vi "CLC_GEN4_L2_InPhaseCal.vi"() -> ()   [LabVIEW 2023, in "Clover_Cell.lvlib"]
uses:
  Clover_Cell.lvlib
  lib/Anritsu Signal Analyzer Series/Anritsu Signal Analyzer Series.lvlib
  lib/ELTA/ELTA.lvlib
  <vilib>/Utility/file.llb/Write Delimited Spreadsheet (DBL).vi
panel:
  out "Check Ref. Ch.":i32[][](array[numeric])
  in  "Dual_Ch.???":bool=TRUE
  in  "Single_Channel_Phase_Sweep":bool
  in  "Polarity":u16(ring) items=["V", "H"]
  in  "AvgTimes":i32=3
  in  "TRXmode":u16(ring)=1 items=["Rx"=2, "Tx"=1]
  in  "CenterFreq(GHz)":dbl=27.0
  in  "VISA resource name":refnum<visa-resource-name>="TCPIP0::192.168.100.230::inst0::INSTR"
  out "Channel":i32=63
  out "Operating \nChannel(s)":bool[][](array[boolean])
  out "FileNAME_Dual":string
  out "FileNAME_Single":string
  out "PhaseStep":i32=63
  out "OK?":bool
  out "output cluster":T1={"address"="192.168.100.111", "remote port or service name"=5025, "timeout ms (60000)"=10000}
  out "SA1":dbl[](graph)
  out "trmode":u16=1
  out "TotalTime":dbl format="%.2f"
  out "StopTime":timestamp=timestamp(3663835912.033212 s since 1904-01-01)
  out "Data":dbl[][](array[numeric])
  out "StartTime":timestamp=timestamp(3663835741.875155 s since 1904-01-01)
  out "error out":errorcluster
  out "CurrentData":dbl[](array[numeric])
  out "Duration":dbl
  # "Setting"
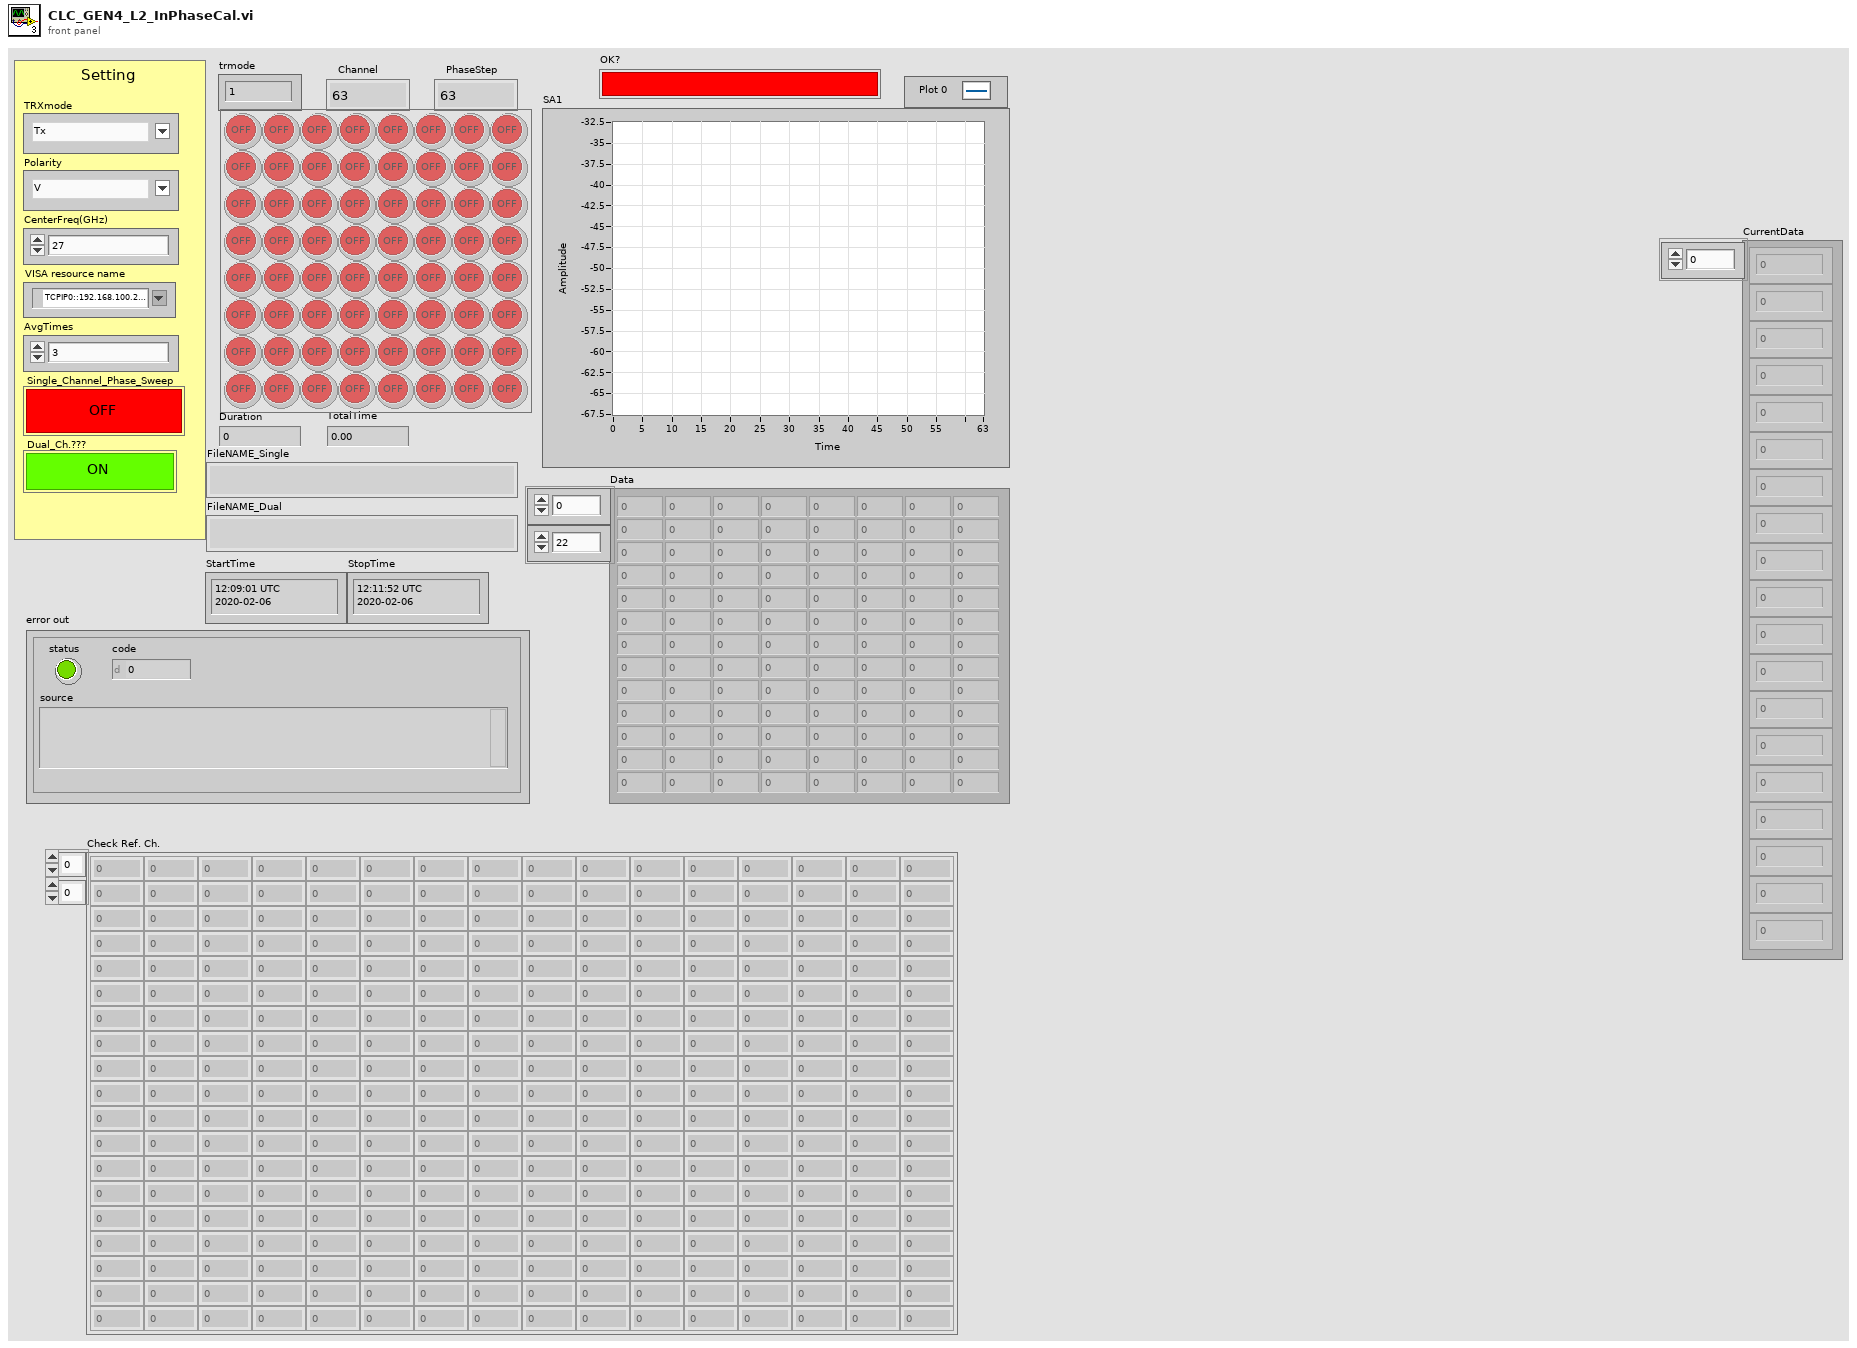
[diagram p1: front panel]
types:
  T1 = cluster{"address":string, "remote port or service name":u16, "timeout ms (60000)":i32}
  T2 = cluster{"Mode":u16, "Polarity":u16, "CH_ON/OFF":u16, "Channel":i32, "Gain":i32, "Phase":i32}
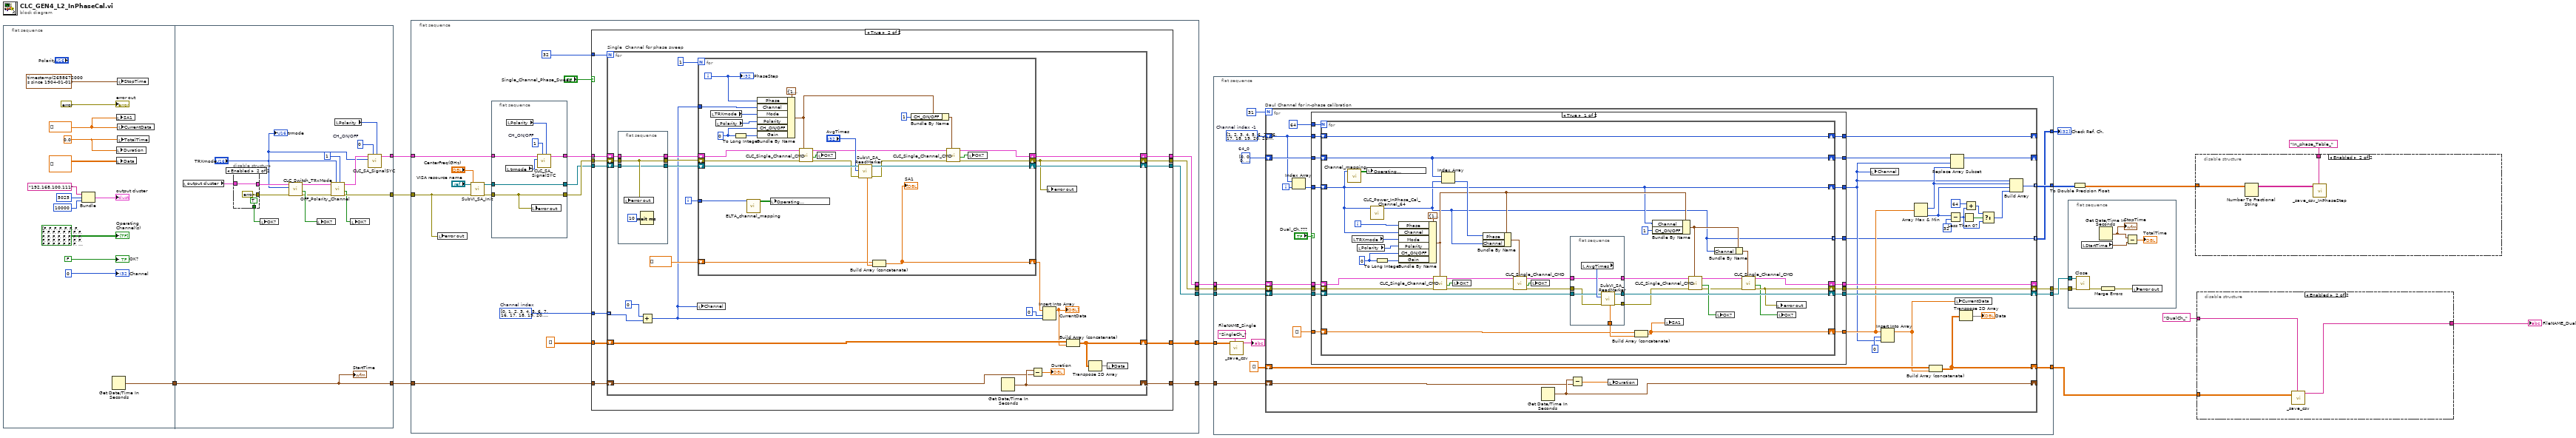
[diagram p0: block diagram]
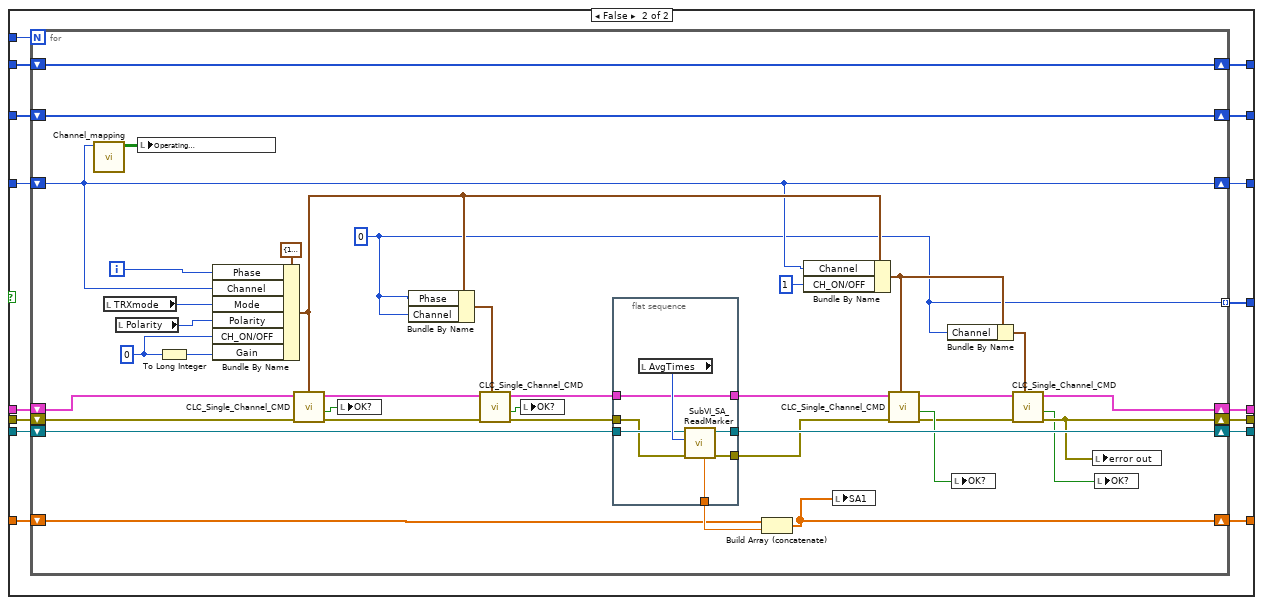
[diagram p2: hidden frame]
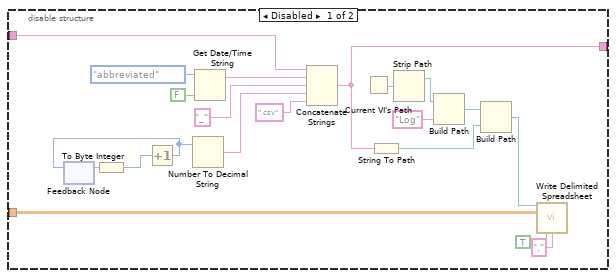
[diagram p4: hidden frame]
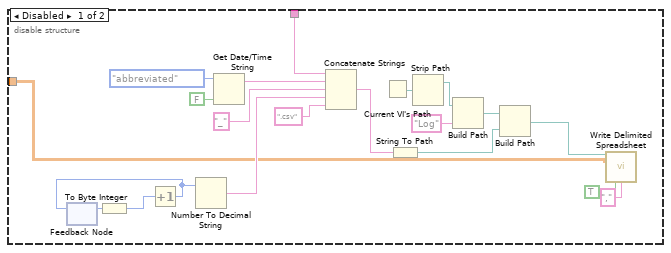
[diagram p5: hidden frame]
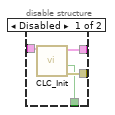
[diagram p6: hidden frame]
diagram:
  n1 = flat-sequence {
    tunnel: [w19] -> w4
    tunnel: w4 -> [w35]
    tunnel: [w38] -> w5
    tunnel: [w42] -> w8
    tunnel: [w35] -> w18
    frame #0 {
      w23 = dbl[] []
      w26 = 0.0 ("TotalTime")
      n2 = Bundle("address"="192.168.100.111", "remote port or service name"=u16 5025, "timeout ms (60000)"=10000) -> (→"output cluster":T1)  [unwired: 1 in]
      n3 = Get Date/Time In Seconds() -> (seconds since 1Jan1904=w19:timestamp)
      n4 = local write "SA1"(w23) -> ()
      n5 = local write "Duration"(w26) -> ()
      n6 = local write "Data"(dbl[][] []) -> ()
      n7 = local write "StopTime"(timestamp(2658672000.001 s since 1904-01-01) ("StopTime")) -> ()
      n8 = local write "CurrentData"(w23) -> ()
      n9 = local write "TotalTime"(w26) -> ()
      "error out" <- errorcluster {"status"=FALSE, "code"=0, "source"=""} ("error out")
      "Operating \nChannel(s)" <- bool[][] [[FALSE, FALSE, FALSE, FALSE, FALSE, FALSE, FALSE, FALSE], [FALSE, FALSE, FALSE, FALSE, FALSE, FALSE, FALSE, FALSE], [FALSE, FALSE, FALSE, FALSE, FALSE, FALSE, FALSE, FALSE], [FALSE, FALSE, FALSE, FALSE, FALSE, FALSE, FALSE, FALSE], [FALSE, FALSE, FALSE, FALSE, FALSE, FALSE, FALSE, FALSE], [FALSE, FALSE, FALSE, FALSE, FALSE, FALSE, FALSE, FALSE], [FALSE, FALSE, FALSE, FALSE, FALSE, FALSE, FALSE, FALSE], [FALSE, FALSE, FALSE, FALSE, FALSE, FALSE, FALSE, FALSE]] ("Operating \nChannel(s)")
      "Channel" <- 0 ("Channel")
      "OK?" <- FALSE ("OK?")
    }
    frame #1 {
      w37 = u16 0  # CH_ON/OFF
      n10 = local read "output cluster"() -> (w47:T1)
      n11 = disable-structure shown="Enabled" {
        disable-tunnel: w47 -> [w51 w54]
        disable-tunnel: [w50 w54] -> w46
        disable-tunnel: [w49 errorcluster {"status"=FALSE, "code"=0, "source"=""} ("error in (no error)")] -> w44
        disable-tunnel: [w48 TRUE ("OK?")] -> w36
        frame Disabled {
          n12 = call "CLC_Init.vi"("TCPIPin"=w51) -> ("error out"=w49:errorcluster, "Status"=w48:bool, "TCPIPin 2"=w50:T1)  [unwired: 8 in]
        }
        frame Enabled {
        }
      }
      n13 = local write "OK?"(w36) -> ()
      n14 = call "CLC_Switch_TRxMode.vi"("error in (no error)"=w44, "Text Ring"="TRXmode", "TCPIPin"=w46) -> ("error out"=w43:errorcluster, "OK?"=w45:bool, "TCPIPin 2"=w41:T1)  [unwired: 6 in]
      n15 = local write "OK?"(w45) -> ()
      n16 = call "OFF_Polarity_Channel.vi"("CH_ON:0/OFF:1"=u16 1, "Mode"="TRXmode", "error in"=w43, "TCPIPin"=w41) -> ("error out"=w42:errorcluster, "OK?"=w40:bool, "TCPIPout"=w39:T1)  [unwired: 5 in]
      n17 = local read "Polarity"() -> (w33:u16)
      n18 = local write "OK?"(w40) -> ()
      n19 = call "CLC_SA_SignalSYC.vi"("Polarity"=w33, "CH_ON/OFF"=w37, "Mode"="TRXmode", "TCPIPin"=w39) -> ("TCPIPout"=w38:T1)  [unwired: 7 in]
      "StartTime" <- w35
      "trmode" <- "TRXmode"
    }
  }
  n20 = flat-sequence {
    tunnel: w18 -> [w71]
    tunnel: [w70] -> w17
    tunnel: [w69] -> w16
    tunnel: [w68] -> w15
    tunnel: [w67] -> w9
    tunnel: w8 -> [w65]
    tunnel: w5 -> [w60]
    tunnel: [w55] -> w3
    frame #0 {
      w62 = i32[] [0, 1, 2, 3, 4, 5, 6, 7, 16, 17, 18, 19, 20, 21, 22, 23, 32, 33, 34, 35, 36, 37, 38, 39, 48, 49, 50, 51, 52, 53, 54, 55]  # Channel index
      n21 = local write "error out"(w65) -> ()
      n22 = call "SubVI_SA_Init.vi"("error in (no error)"=w65, "CenterFreq(GHz) 2"="CenterFreq(GHz)", "VISA resource name"="VISA resource name") -> ("error out 2"=w66:errorcluster, "VISA resource name out"=w59:refnum<visa-resource-name>)  [unwired: 6 in, 1 out]
      n23 = flat-sequence {
        tunnel: w66 -> [w152]
        tunnel: [w152] -> w61
        tunnel: w60 -> [w150]
        tunnel: w59 -> [w151]
        tunnel: [w151] -> w58
        tunnel: [w149] -> w57
        frame #0 {
          w148 = u16 1  # CH_ON/OFF
          n24 = local read "trmode"() -> (w146:u16)
          n25 = local read "Polarity"() -> (w147:u16)
          n26 = local write "error out"(w152) -> ()
          n27 = call "CLC_SA_SignalSYC.vi"("Polarity"=w147, "CH_ON/OFF"=w148, "Mode"=w146, "TCPIPin"=w150) -> ("TCPIPout"=w149:T1)  [unwired: 7 in]
        }
      }
      n28 = case shown="True" "Single_Channel_Phase_Sweep" {
        tunnel: [w75 w90] -> w55
        tunnel: 32 -> [_ w89]
        tunnel: w71 -> [w74 w88]
        tunnel: [w76 w87] -> w70
        tunnel: [w77 w86] -> w69
        tunnel: [w78 w85] -> w68
        tunnel: [w74 w84] -> w67
        tunnel: dbl[][] [] -> [w75 w83]
        tunnel: w62 -> [_ w82]
        tunnel: w61 -> [w77 w81]
        tunnel: w58 -> [w76 w80]
        tunnel: w57 -> [w78 w79]
        frame False {
        }
        frame True {
          n29 = for "Single  Channel for phase sweep" {
            N: w89 -> [_]
            shift-right: [w114] -> w85
            shift-left: w79 -> [w98]
            shift-right: [w108] -> w86
            shift-left: w81 -> [w100]
            shift-right: [w112] -> w87
            shift-left: w80 -> [w97]
            shift-right: [w106] -> w90
            shift-left: w83 -> [w107]
            shift-right: [w110] -> w84
            shift-left: w88 -> [w109]
            tunnel: w82 -> [w94] mode=indexing
            i -> [w93]
            n30 = flat-sequence {
              tunnel: [w116] -> w96
              tunnel: w100 -> [w117]
              tunnel: [w117] -> w99
              tunnel: w98 -> [w116]
              tunnel: w97 -> [w115]
              tunnel: [w115] -> w95
              frame #0 {
                n31 = local write "error out"(w117) -> ()
                n32 = Wait (ms)(milliseconds to wait=u32 10) -> ()  [unwired: 1 out]
              }
            }
            n33 = Add(x=0, y=w94) -> (x+y=w92:i32)
            n34 = local write "Channel"(w92) -> ()
            n35 = for {
              N: 1 -> [_]
              shift-right: [w125] -> w114
              shift-left: w96 -> [w137]
              shift-right: [w127] -> w108
              shift-left: w99 -> [w139]
              shift-right: [w144] -> w112
              shift-left: w95 -> [w145]
              shift-right: [w140] -> w105
              shift-left: dbl[] [] -> [w141]
              tunnel: w92 -> [w134]
              tunnel: w93 -> [w120]
              i -> [w130]
              w131 = u16 0 ("CH_ON/OFF")
              n36 = local read "TRXmode"() -> (w133:u16)
              n37 = local read "Polarity"() -> (w132:u16)
              n38 = To Long Integer(number=w131) -> (32bit integer=w129:i32)
              n39 = call "ELTA_channel_mapping.vi"("Channel IN"=w120) -> ("Operating \nChannel(s)"=w119:bool[][])  [unwired: 10 in]
              n40 = Bundle By Name(cluster=T2 {"Mode"=1, "Polarity"=1, "CH_ON/OFF"=1, "Channel"=0, "Gain"=0, "Phase"=0} ("Channel params"), "Phase"=w130, "Channel"=w134, "Mode"=w133, "Polarity"=w132, "CH_ON/OFF"=w131, "Gain"=w129) -> (w124:T2)
              n41 = local write "Operating \nChannel(s)"(w119) -> ()
              n42 = call "CLC_Single_Channel_CMD.vi"("Channel params"=w124, "error in"=w139, "TCPIPin"=w137) -> ("error out"=w138:errorcluster, "OK?"=w135:bool, "TCPIPout"=w126:T1)  [unwired: 6 in]
              n43 = local write "OK?"(w135) -> ()
              n44 = call "SubVI_SA_ReadMarker.vi"("error in (no error)"=w138, "AvgTimes"="AvgTimes", "VISA resource name"=w145) -> ("error out"=w128:errorcluster, "VISA resource name out"=w144:refnum<visa-resource-name>, "Marker Power"=w142:dbl)  [unwired: 5 in, 1 out]
              n45 = Build Array (concatenate)(w141, w142) -> (w140:dbl[])
              "SA1" <- w140
              n46 = Bundle By Name(cluster=w124, "CH_ON/OFF"=u16 1) -> (w122:T2)
              n47 = call "CLC_Single_Channel_CMD.vi"("Channel params"=w122, "error in"=w128, "TCPIPin"=w126) -> ("error out"=w127:errorcluster, "OK?"=w121:bool, "TCPIPout"=w125:T1)  [unwired: 6 in]
              n48 = local write "OK?"(w121) -> ()
              "PhaseStep" <- w130
            }
            n49 = Get Date/Time In Seconds() -> (seconds since 1Jan1904=w110:timestamp)
            n50 = Subtract(x=w110, y=w109) -> (x-y=→"Duration":dbl)
            n51 = Insert Into Array(array=w105, index=0, new element=w92) -> (w102:dbl[])
            "CurrentData" <- w102
            n52 = local write "error out"(w108) -> ()
            n53 = Build Array (concatenate)(w107, w102) -> (w106:dbl[][])
            n54 = Transpose 2D Array(2D array=w106) -> (transposed array=w91:dbl[][])
            n55 = local write "Data"(w91) -> ()
          }
        }
      }
    }
  }
  n56 = flat-sequence {
    tunnel: w17 -> [w167]
    tunnel: w16 -> [w166]
    tunnel: w15 -> [w165]
    tunnel: [w164] -> w12
    tunnel: [w163] -> w11
    tunnel: [w162] -> w10
    tunnel: w9 -> [w161]
    tunnel: [w159] -> w6
    tunnel: w3 -> [w157]
    tunnel: [w153] -> w1
    frame #0 {
      w154 = i32[] [0, 0, 0, 0, 0, 0, 0, 0, 0, 0, 0, 0, 0, 0, 0, 0, 0, 0, 0, 0, 0, 0, 0, 0, 0, 0, 0, 0, 0, 0, 0, 0, 0, 0, 0, 0, 0, 0, 0, 0, 0, 0, 0, 0, 0, 0, 0, 0, 0, 0, 0, 0, 0, 0, 0, 0, 0, 0, 0, 0, 0, 0, 0, 0]  # 64_0
      w158 = i32[] [1, 2, 3, 4, 5, 6, 7, 16, 17, 18, 19, 20, 21, 22, 23, 32, 33, 34, 35, 36, 37, 38, 39, 48, 49, 50, 51, 52, 53, 54, 55]  # Channel index -1
      n57 = call "_save_csv.vi"("delimiter (\\t)"="SingleCh_" ("delimiter (\\t)"), "Data"=w157) -> ("FileName"=→"FileNAME_Single":string)  [unwired: 9 in]
      n58 = for "Daul Channel for in-phase calibration" {
        N: 31 -> [_]
        shift-right: [w204] -> _
        shift-left: w165 -> [w189]
        shift-right: [w201] -> w162
        shift-left: w166 -> [w190]
        shift-right: [w202] -> w163
        shift-left: w167 -> [w200]
        shift-right: [w195] -> w164
        shift-left: dbl[][] [] -> [w196]
        shift-right: [w199] -> _
        shift-left: w161 -> [w198]
        shift-right: [w173] -> _
        shift-left: w154 -> [w185]
        tunnel: [w187] -> w159 mode=indexing
        shift-right: [w184] -> _
        shift-left: w158 -> [w183]
        tunnel: [w169] -> w153 mode=indexing
        i -> [w186]
        n59 = Index Array(array=w183, index=w186) -> (element=w182:i32)
        n60 = case shown="True" "Dual_Ch.???" {
          tunnel: [w220 w281] -> w204
          tunnel: 64 -> [w219 w280]
          tunnel: [w218 w279] -> w202
          tunnel: [w217 w278] -> w201
          tunnel: w200 -> [w216 w277]
          tunnel: dbl[] [] -> [w215 w276]
          tunnel: w190 -> [w214 w275]
          tunnel: w189 -> [w213 w274]
          tunnel: [w212 w273] -> w188
          tunnel: w185 -> [w211 w272]
          tunnel: [w210 w271] -> w184
          tunnel: w183 -> [w209 w270]
          tunnel: w182 -> [w208 w269]
          tunnel: [w207 w268] -> w174
          tunnel: [w206 w267] -> w171
          tunnel: [w205 w266] -> w169
          frame True {
            n61 = for {
              N: w219 -> [_]
              shift-right: [w227] -> w220
              shift-left: w213 -> [w247]
              shift-right: [w232] -> w217
              shift-left: w214 -> [w249]
              shift-right: [w258] -> w218
              shift-left: w216 -> [w255]
              shift-right: [w223] -> w212
              shift-left: w215 -> [w256]
              shift-right: [w240] -> w207
              shift-left: w211 -> [w240]
              shift-right: [w225] -> w210
              shift-left: w209 -> [w225]
              shift-right: [w222] -> w206
              shift-left: w208 -> [w222]
              tunnel: [w221] -> w205 mode=indexing
              i -> [w248]
              w253 = u16 0 ("CH_ON/OFF")
              n62 = call "Channel_mapping.vi"("Channel IN"=w222) -> ("Operating \nChannel(s)"=w226:bool[][])  [unwired: 10 in]
              n63 = local read "TRXmode"() -> (w251:u16)
              n64 = local read "Polarity"() -> (w252:u16)
              n65 = local write "Operating \nChannel(s)"(w226) -> ()
              n66 = call "CLC_Power_InPhase_Cal_Channel_64.vi"("Channel IN"=w222) -> ("Ref_Channel"=w221:i32)  [unwired: 8 in, 2 out]
              n67 = To Long Integer(number=w253) -> (32bit integer=w254:i32)
              n68 = Bundle By Name(cluster=T2 {"Mode"=1, "Polarity"=1, "CH_ON/OFF"=1, "Channel"=0, "Gain"=0, "Phase"=0} ("Channel params"), "Phase"=w248, "Channel"=w222, "Mode"=w251, "Polarity"=w252, "CH_ON/OFF"=w253, "Gain"=w254) -> (w230:T2)
              n69 = call "CLC_Single_Channel_CMD.vi"("Channel params"=w230, "error in"=w249, "TCPIPin"=w247) -> ("error out"=w245:errorcluster, "OK?"=w244:bool, "TCPIPout"=w246:T1)  [unwired: 6 in]
              n70 = Index Array(array=w240, index=w221) -> (element=w239:i32)
              n71 = local write "OK?"(w244) -> ()
              n72 = Bundle By Name(cluster=w230, "Phase"=w239, "Channel"=w221) -> (w243:T2)
              n73 = call "CLC_Single_Channel_CMD.vi"("Channel params"=w243, "error in"=w245, "TCPIPin"=w246) -> ("error out"=w241:errorcluster, "OK?"=w242:bool, "TCPIPout"=w238:T1)  [unwired: 6 in]
              n74 = local write "OK?"(w242) -> ()
              n75 = flat-sequence {
                tunnel: [w265] -> w258
                tunnel: [w263] -> w257
                tunnel: [w262] -> w237
                tunnel: w255 -> [w261]
                tunnel: w241 -> [w260]
                tunnel: [w259] -> w236
                tunnel: w238 -> [w259]
                frame #0 {
                  n76 = local read "AvgTimes"() -> (w264:i32)
                  n77 = call "SubVI_SA_ReadMarker.vi"("error in (no error)"=w260, "AvgTimes"=w264, "VISA resource name"=w261) -> ("error out"=w262:errorcluster, "VISA resource name out"=w265:refnum<visa-resource-name>, "Marker Power"=w263:dbl)  [unwired: 5 in, 1 out]
                }
              }
              n78 = Build Array (concatenate)(w256, w257) -> (w223:dbl[])
              n79 = Bundle By Name(cluster=w230, "Channel"=w222, "CH_ON/OFF"=u16 1) -> (w224:T2)
              n80 = local write "SA1"(w223) -> ()
              n81 = call "CLC_Single_Channel_CMD.vi"("Channel params"=w224, "error in"=w237, "TCPIPin"=w236) -> ("error out"=w233:errorcluster, "OK?"=w234:bool, "TCPIPout"=w231:T1)  [unwired: 6 in]
              n82 = Bundle By Name(cluster=w224, "Channel"=w221) -> (w229:T2)
              n83 = local write "OK?"(w234) -> ()
              n84 = call "CLC_Single_Channel_CMD.vi"("Channel params"=w229, "error in"=w233, "TCPIPin"=w231) -> ("error out"=w232:errorcluster, "OK?"=w228:bool, "TCPIPout"=w227:T1)  [unwired: 6 in]
              n85 = local write "error out"(w232) -> ()
              n86 = local write "OK?"(w228) -> ()
            }
          }
          frame False {
            n87 = for {
              N: w280 -> [_]
              shift-right: [w288] -> w281
              shift-left: w274 -> [w307]
              shift-right: [w293] -> w278
              shift-left: w275 -> [w309]
              shift-right: [w318] -> w279
              shift-left: w277 -> [w315]
              shift-right: [w284] -> w273
              shift-left: w276 -> [w316]
              shift-right: [w300] -> w268
              shift-left: w272 -> [w300]
              shift-right: [w286] -> w271
              shift-left: w270 -> [w286]
              shift-right: [w283] -> w267
              shift-left: w269 -> [w283]
              tunnel: [w282] -> w266 mode=indexing
              i -> [w308]
              w282 = 0 ("Ref_Channel")
              w313 = u16 0 ("CH_ON/OFF")
              n88 = call "Channel_mapping.vi"("Channel IN"=w283) -> ("Operating \nChannel(s)"=w287:bool[][])  [unwired: 10 in]
              n89 = local read "TRXmode"() -> (w311:u16)
              n90 = local read "Polarity"() -> (w312:u16)
              n91 = local write "Operating \nChannel(s)"(w287) -> ()
              n92 = To Long Integer(number=w313) -> (32bit integer=w314:i32)
              n93 = Bundle By Name(cluster=T2 {"Mode"=1, "Polarity"=1, "CH_ON/OFF"=1, "Channel"=0, "Gain"=0, "Phase"=0} ("Channel params"), "Phase"=w308, "Channel"=w283, "Mode"=w311, "Polarity"=w312, "CH_ON/OFF"=w313, "Gain"=w314) -> (w291:T2)
              n94 = call "CLC_Single_Channel_CMD.vi"("Channel params"=w291, "error in"=w309, "TCPIPin"=w307) -> ("error out"=w305:errorcluster, "OK?"=w304:bool, "TCPIPout"=w306:T1)  [unwired: 6 in]
              n95 = local write "OK?"(w304) -> ()
              n96 = Bundle By Name(cluster=w291, "Phase"=w282, "Channel"=w282) -> (w303:T2)
              n97 = call "CLC_Single_Channel_CMD.vi"("Channel params"=w303, "error in"=w305, "TCPIPin"=w306) -> ("error out"=w301:errorcluster, "OK?"=w302:bool, "TCPIPout"=w299:T1)  [unwired: 6 in]
              n98 = local write "OK?"(w302) -> ()
              n99 = flat-sequence {
                tunnel: [w325] -> w318
                tunnel: [w323] -> w317
                tunnel: [w322] -> w298
                tunnel: w315 -> [w321]
                tunnel: w301 -> [w320]
                tunnel: [w319] -> w297
                tunnel: w299 -> [w319]
                frame #0 {
                  n100 = local read "AvgTimes"() -> (w324:i32)
                  n101 = call "SubVI_SA_ReadMarker.vi"("error in (no error)"=w320, "AvgTimes"=w324, "VISA resource name"=w321) -> ("error out"=w322:errorcluster, "VISA resource name out"=w325:refnum<visa-resource-name>, "Marker Power"=w323:dbl)  [unwired: 5 in, 1 out]
                }
              }
              n102 = Build Array (concatenate)(w316, w317) -> (w284:dbl[])
              n103 = Bundle By Name(cluster=w291, "Channel"=w283, "CH_ON/OFF"=u16 1) -> (w285:T2)
              n104 = local write "SA1"(w284) -> ()
              n105 = call "CLC_Single_Channel_CMD.vi"("Channel params"=w285, "error in"=w298, "TCPIPin"=w297) -> ("error out"=w294:errorcluster, "OK?"=w295:bool, "TCPIPout"=w292:T1)  [unwired: 6 in]
              n106 = Bundle By Name(cluster=w285, "Channel"=w282) -> (w290:T2)
              n107 = local write "OK?"(w295) -> ()
              n108 = call "CLC_Single_Channel_CMD.vi"("Channel params"=w290, "error in"=w294, "TCPIPin"=w292) -> ("error out"=w293:errorcluster, "OK?"=w289:bool, "TCPIPout"=w288:T1)  [unwired: 6 in]
              n109 = local write "error out"(w293) -> ()
              n110 = local write "OK?"(w289) -> ()
            }
          }
        }
        n111 = Get Date/Time In Seconds() -> (seconds since 1Jan1904=w199:timestamp)
        n112 = Subtract(x=w199, y=w198) -> (x-y=w197:dbl)
        n113 = local write "Duration"(w197) -> ()
        n114 = local write "Channel"(w171) -> ()
        n115 = Insert Into Array(array=w188, index=0, new element=w171) -> (w191:dbl[])
        n116 = Array Max & Min(array=w188) -> (max index (indices)=w172:i32, min index (indices)=w181:i32)  [unwired: 2 out]
        n117 = Build Array (concatenate)(w196, w191) -> (w195:dbl[][])
        n118 = Subtract(x=w181, y=32) -> (x-y=w176:i32)
        n119 = Replace Array Subset(array=w174, new element=w172, index=w171) -> (w173:i32[])
        n120 = local write "CurrentData"(w191) -> ()
        n121 = Transpose 2D Array(2D array=w195) -> (transposed array=→"Data":dbl[][])
        n122 = Less Than 0?(x=w176) -> (x < 0?=w179:bool)
        n123 = Add(x=64, y=w176) -> (x+y=w177:i32)
        n124 = Select(t=w177, s=w179, f=w176) -> (s? t:f=w175:i32)
        n125 = Build Array(w171, w172, w181, w175) -> (w187:i32[])
      }
    }
  }
  n126 = flat-sequence {
    tunnel: w11 -> [w331]
    tunnel: w10 -> [w330]
    frame #0 {
      n127 = call "Close.vi"("error in (no error)"=w330, "VISA resource name"=w331) -> ("error out"=w332:errorcluster)  [unwired: 9 in]
      n128 = local read "StartTime"() -> (w326:timestamp)
      n129 = Get Date/Time In Seconds() -> (seconds since 1Jan1904=w327:timestamp)
      "StopTime" <- w327
      n130 = Merge Errors(w332) -> (w329:errorcluster)
      n131 = Subtract(x=w327, y=w326) -> (x-y=→"TotalTime":dbl)
      n132 = local write "error out"(w329) -> ()
    }
  }
  n133 = To Double Precision Float(number=w6) -> (double precision float=w2:dbl[][])
  n134 = disable-structure shown="Enabled" {
    disable-tunnel: "In_phase_Table_" ("delimiter (\\t)") -> [w342 w354]
    disable-tunnel: w2 -> [w334 w355]
    frame Disabled {
      n135 = feedback #1() -> (w343:i8)  [unwired: 1 in]
      n136 = To Byte Integer(number=w343) -> (8bit integer=w345:i8)
      n137 = Increment(x=w345) -> (x+1=w344:i8)
      n138 = feedback-in #1(w344) -> ()
      n139 = Number To Decimal String(number=w344) -> (decimal integer string=w346:string)  [unwired: 1 in]
      n140 = Get Date/Time String(date format (0)=enum16{"short", "long", "abbreviated"}."abbreviated", want seconds? (F)=FALSE) -> (date string=w337:string)  [unwired: 1 in, 1 out]
      n141 = Concatenate Strings(w342, w337, "_" ("delimiter (\\t)"), w346, ".csv" ("delimiter (\\t)")) -> (w338:string)
      n142 = Current VI's Path() -> (path=w351:path)
      n143 = String To Path(string=w338) -> (path=w352:path)
      n144 = Strip Path(path=w351) -> (stripped path=w350:path)  [unwired: 1 out]
      n145 = Build Path(base path=w350, name or relative path="Log") -> (appended path=w348:path)
      n146 = Build Path(base path=w348, name or relative path=w352) -> (appended path=w333:path)
      n147 = call-poly <vilib>:"Write Delimited Spreadsheet.vi"("file path (dialog if empty)"=w333, "2D data"=w334, "transpose? (no:F)"=TRUE, "delimiter (\\t)"="," ("delimiter (\\t)")) -> ()  [unwired: 10 in, 2 out]
    }
    frame Enabled {
      n148 = Number To Fractional String(number=w355) -> (F-format string=w353:string[][])  [unwired: 3 in]
      n149 = call "_save_csv_InPhaseStep.vi"("delimiter (\\t)"=w354, "dataInput"=w353) -> ()  [unwired: 9 in, 1 out]
    }
  }
  n150 = disable-structure shown="Enabled" {
    disable-tunnel: [w374 w376] -> w14
    disable-tunnel: "DualCh_" ("delimiter (\\t)") -> [w370 w377]
    disable-tunnel: w12 -> [w369 w378]
    frame Disabled {
      n151 = feedback #2() -> (w368:i8)  [unwired: 1 in]
      n152 = To Byte Integer(number=w368) -> (8bit integer=w366:i8)
      n153 = Increment(x=w366) -> (x+1=w367:i8)
      n154 = feedback-in #2(w367) -> ()
      n155 = Number To Decimal String(number=w367) -> (decimal integer string=w365:string)  [unwired: 1 in]
      n156 = Get Date/Time String(date format (0)=enum16{"short", "long", "abbreviated"}."abbreviated", want seconds? (F)=FALSE) -> (date string=w375:string)  [unwired: 1 in, 1 out]
      n157 = Concatenate Strings(w370, w375, "_" ("delimiter (\\t)"), w365, ".csv" ("delimiter (\\t)")) -> (w374:string)
      n158 = Current VI's Path() -> (path=w360:path)
      n159 = String To Path(string=w374) -> (path=w359:path)
      n160 = Strip Path(path=w360) -> (stripped path=w361:path)  [unwired: 1 out]
      n161 = Build Path(base path=w361, name or relative path="Log") -> (appended path=w363:path)
      n162 = Build Path(base path=w363, name or relative path=w359) -> (appended path=w358:path)
      n163 = call-poly <vilib>:"Write Delimited Spreadsheet.vi"("file path (dialog if empty)"=w358, "2D data"=w369, "transpose? (no:F)"=TRUE, "delimiter (\\t)"="," ("delimiter (\\t)")) -> ()  [unwired: 10 in, 2 out]
    }
    frame Enabled {
      n164 = call "_save_csv.vi"("delimiter (\\t)"=w377, "Data"=w378) -> ("FileName"=w376:string)  [unwired: 9 in]
    }
  }
  "FileNAME_Dual" <- w14
  "Check Ref. Ch." <- w1
